vi "Mood Features.vi"(0 "Mic Input":waveform(dbl)[](array[waveform]), 1 "Sampling rate":dbl=32000.0 format="%#_13g") -> (2 "PSD":cluster{"f0":dbl, "df":dbl, "magnitude":dbl[]}[](graph), 3 "Intensity":T1, 4 "Timbre":T3, 5 "Rhythm":T2)   [LabVIEW 2013]
uses:
  <vilib>/measure/maspectr.llb/Power Spectrum and PSD Export Mode.ctl
  <vilib>/Analysis/4window.llb/windowTd.ctl
  <vilib>/measure/maspectr.llb/FFT Power Spectrum and PSD for N Chan.vi
  <vilib>/measure/NI_MAPro.lvlib
  <vilib>/Analysis/NI_AALPro.lvlib
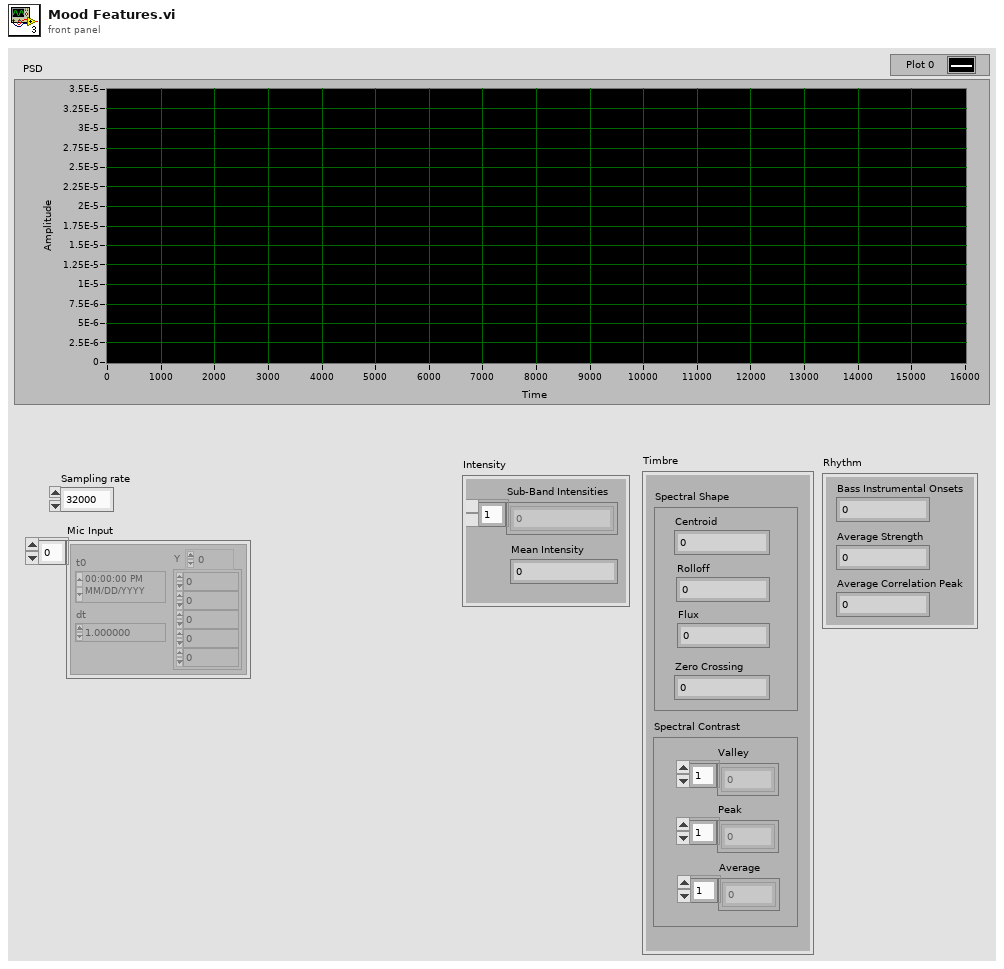
[diagram p1: front panel]
types:
  T1 = cluster{"Sub-Band Intensities":dbl[], "Mean Intensity":dbl}
  T2 = cluster{"Bass Instrumental Onsets":i32, "Average Strength":dbl, "Average Correlation Peak":dbl}
  T3 = cluster{"Spectral Shape":cluster{"Centroid":dbl, "Rolloff":dbl, "Flux":dbl, "Zero Crossing":dbl}, "Spectral Contrast":cluster{"Valley":dbl[], "Peak":dbl[], "Average":dbl[]}}
  T4 = typedef "NI_AALPro.lvlib/windowTd.ctl" = u32
  T5 = typedef "NI_MAPro.lvlib/Power Spectrum and PSD Export Mode.ctl" = u16
  T6 = cluster{"Power Spectrum / PSD[0]":cluster{"f0":dbl, "df":dbl, "magnitude":dbl[]}, "Power Spectrum / PSD[1]":cluster{"f0":dbl, "df":dbl, "magnitude":dbl[]}, "Power Spectrum / PSD[2]":cluster{"f0":dbl, "df":dbl, "magnitude":dbl[]}, "Power Spectrum / PSD[3]":cluster{"f0":dbl, "df":dbl, "magnitude":dbl[]}, "Power Spectrum / PSD[4]":cluster{"f0":dbl, "df":dbl, "magnitude":dbl[]}, "Power Spectrum / PSD[5]":cluster{"f0":dbl, "df":dbl, "magnitude":dbl[]}, "Power Spectrum / PSD[6]":cluster{"f0":dbl, "df":dbl, "magnitude":dbl[]}, "Power Spectrum / PSD[7]":cluster{"f0":dbl, "df":dbl, "magnitude":dbl[]}, "Power Spectrum / PSD[8]":cluster{"f0":dbl, "df":dbl, "magnitude":dbl[]}}
  T7 = cluster{"Sub_Band Valley":dbl[], "Sub-Band Peak":dbl[], "Sub-Band Average":dbl[]}
  T8 = cluster{"Spectral Centroid":dbl, "Spectral Rolloff":dbl, "Spectral Flux":dbl, "Zero Crossing":dbl}
  T9 = cluster{cluster{"Spectral Centroid":dbl, "Spectral Rolloff":dbl, "Spectral Flux":dbl, "Zero Crossing":dbl}, cluster{"Sub_Band Valley":dbl[], "Sub-Band Peak":dbl[], "Sub-Band Average":dbl[]}}
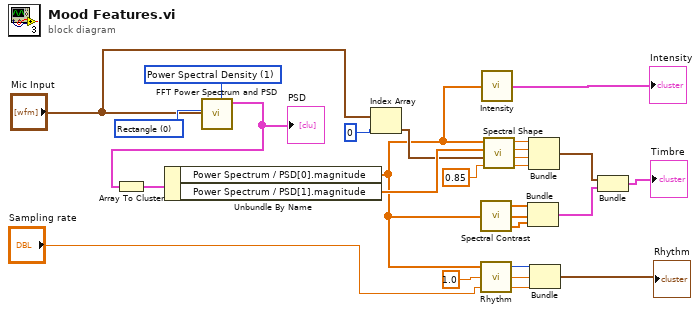
[diagram p0: block diagram]
diagram:
  w26 = T4 0 items=["Rectangle"=0, "Hanning"=1, "Hamming"=2, "Blackman-Harris"=3, "Exact Blackman"=4, "Blackman"=5, "Flat Top"=6, "4 Term B-Harris "=7, "7 Term B-Harris"=8, "Low Sidelobe"=9, "Blackman Nuttall"=11, "Triangle"=30, "Bartlett-Hanning"=31, "Bohman"=32, "Parzen"=33, "Welch"=34, "Kaiser"=60, "Dolph-Chebyshev"=61, "Gaussian"=62] ("window")
  w27 = T5 1 items=["Power Spectrum", "Power Spectral Density"] ("export mode")
  n1 = call-poly <vilib>:"FFT Power Spectrum and PSD.vi"("export mode"=w27, "window"=w26, "time signals"="Mic Input") -> ("Power Spectrum / PSD"=w1:cluster{"f0":dbl, "df":dbl, "magnitude":dbl[]}[])  [unwired: 5 in, 3 out]
  "PSD" <- w1
  n2 = Array To Cluster(array=w1) -> (cluster=w25:T6)
  n3 = Unbundle By Name(w25) -> ("Power Spectrum / PSD[0].magnitude"=w2:dbl[], "Power Spectrum / PSD[1].magnitude"=w24:dbl[])
  n4 = Index Array(array="Mic Input", index=0) -> (element=w7:waveform(dbl))
  n5 = call "Spectral Contrast.vi"("Array"=w2) -> ("Sub_Band Valley"=w20:dbl[], "Sub-Band Peak"=w19:dbl[], "Sub-Band Average"=w18:dbl[])
  n6 = call "Rhythm.vi"("Sampling rate"="Sampling rate", "Segment Length"=1.0, "Array"=w2) -> ("Average Correlation Peak"=w11:dbl, "Average Strength"=w12:dbl, "Bass Instrumental Onsets"=w13:i32)
  n7 = call "Intensity.vi"("PSD[0]"=w2) -> ("Intensity"=→"Intensity":T1)
  n8 = call "Spectral Shape.vi"("cutoff"=0.85, "Waveform"=w7, "PSD[1]"=w24, "PSD[0]"=w2) -> ("Zero Crossing"=w4:dbl, "Spectral Rolloff"=w22:dbl, "Spectral Flux"=w21:dbl, "Spectral Centroid"=w23:dbl)
  n9 = Bundle("Sub_Band Valley"=w20, "Sub-Band Peak"=w19, "Sub-Band Average"=w18) -> (w16:T7)  [unwired: 1 in]
  n10 = Bundle("Spectral Centroid"=w23, "Spectral Rolloff"=w22, "Spectral Flux"=w21, "Zero Crossing"=w4) -> (w17:T8)  [unwired: 1 in]
  n11 = Bundle("Bass Instrumental Onsets"=w13, "Average Strength"=w12, "Average Correlation Peak"=w11) -> (→"Rhythm":T2)  [unwired: 1 in]
  n12 = Bundle(w17, w16) -> (→"Timbre":T9)  [unwired: 1 in]
